vi "FinishSequenceADCHannel.vi"(5 "Numeric 2":i32, 10 "error out 2":errorcluster) -> (0 "to shell":string caption="Result", 2 "error out":errorcluster)   [LabVIEW 2009]
uses:
  lib/System Files/user.lib/atmcd32d.llb/HSSpeed_type typedef.ctl
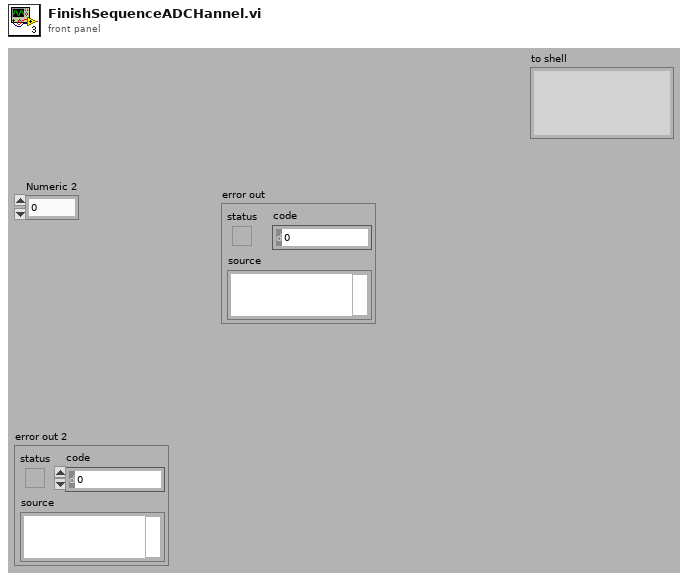
[diagram p1: front panel]
types:
  T1 = typedef "HSSpeed_type typedef.ctl" = enum16{"EM Amp", "Conventional Amp"}
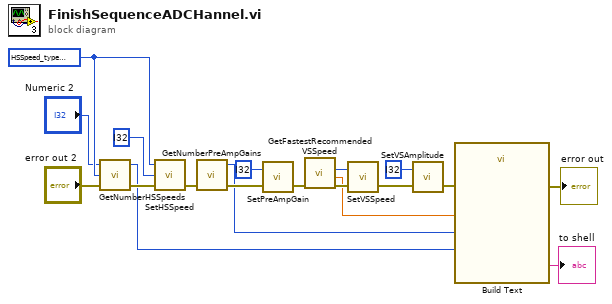
[diagram p0: block diagram]
diagram:
  w19 = T1 ? ("Get#HSSpeedsType")
  n1 = call "GetNumberHSSpeeds.vi"("error in (no error)"="error out 2", "type"=w19, "channel"="Numeric 2") -> ("error out"=w10:errorcluster, "number"=w4:i32)  [unwired: 1 out]
  n2 = call "SetHSSpeed.vi"("error in (no error)"=w10, "index"=i32 ? ("SetHSSpeed"), "type"=w19) -> ("error out"=w7:errorcluster)  [unwired: 1 in, 1 out]
  n3 = call "GetNumberPreAmpGains.vi"("error in (no error)"=w7) -> ("error out"=w8:errorcluster, "number"=w3:i32)  [unwired: 2 in, 1 out]
  n4 = call "SetPreAmpGain.vi"("error in (no error)"=w8, "index"=i32 ? ("SetPreAmpGain")) -> ("error out"=w12:errorcluster)  [unwired: 1 out]
  n5 = call "GetFastestRecommendedVSSpeed.vi"("error in (no error)"=w12) -> ("error out"=w13:errorcluster, "speed"=w2:sgl, "index"=w15:u32)  [unwired: 3 in, 1 out]
  n6 = call "SetVSSpeed.vi"("error in (no error)"=w13, "index"=w15) -> ("error out"=w14:errorcluster)  [unwired: 1 out]
  n7 = call "SetVSAmplitude.vi"("error in (no error)"=w14, "amplitude"=i32 ? ("SetVSAmplit")) -> ("error out"=w6:errorcluster)  [unwired: 1 out]
  n8 = call "Build Text"("vs"=w2, "pregain"=w3, "hs"=w4, "error in (no error)"=w6) -> ("Result"=→"to shell":string, "error out"=→"error out":errorcluster)  [unwired: 10 in]
